vi "Paragraph_CreateStandardText.vi"(10 "error in":errorcluster, 11 "document":refnum<k24>) -> (2 "error out":errorcluster, 3 "StandardTextParagraph":refnum<k24>)   [LabVIEW 2009]
uses:
  C:/Projets/LAVAG/OpenOfficeRGT/AODL/DLLs/AODL.dll
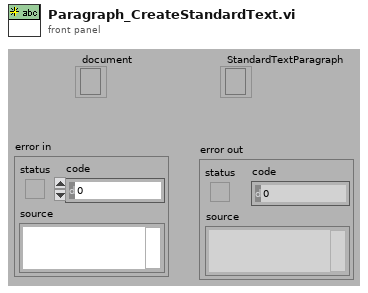
[diagram p1: front panel]
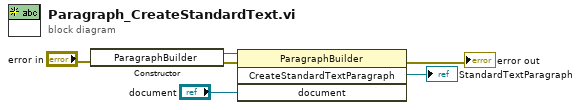
[diagram p0: block diagram]
diagram:
  n1 = constructor class="ParagraphBuilder"(error in="error in") -> (reference out=w5:refnum<k24>, error out=w6:errorcluster)  [unwired: 2 in, 1 out]
  n2 = invoke class="ParagraphBuilder" method="CreateStandardTextParagraph"(reference=w5, error in=w6, "document"="document") -> (error out=→"error out":errorcluster, "CreateStandardTextParagraph"=→"StandardTextParagraph":refnum<k24>)  [unwired: 1 in, 2 out]
